vi "getWaveform.vi"(7 "Chn":string, 8 "error in (no error)":errorcluster, 11 "ScopeNi in":refnum<class "ScopeNi.lvclass">) -> (0 "error out":errorcluster, 2 "Waveform Graph":waveform(dbl)(graph), 3 "ScopeNi out":refnum<class "ScopeNi.lvclass">)   [LabVIEW 2023, in "ScopeNi.lvclass"]
doc: "<b>Author:</b> Wolfgang\n<b>Description:</b> Fetches the waveform for the given channel from the scope."
uses:
  ScopeNi.lvclass
  ScopeNi.lvclass/ScopeNi.ctl
  <instrlib>/niScope/Acquire/Fetch/niScope Fetch WDT.vi
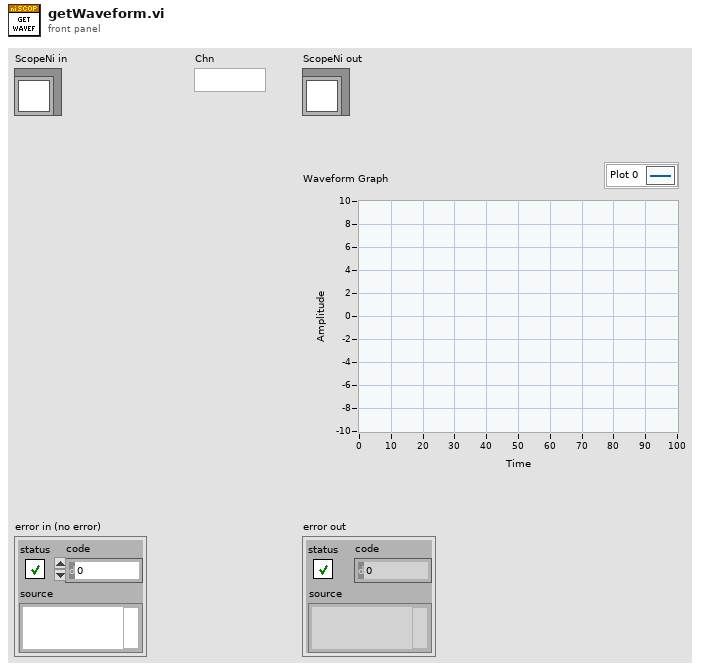
[diagram p1: front panel]
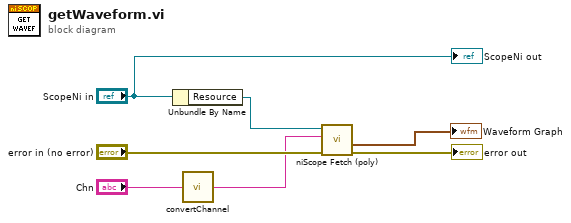
[diagram p0: block diagram]
diagram:
  n1 = Unbundle By Name("ScopeNi in") -> ("Resource"=w5:refnum<k15>)
  n2 = call "convertChannel.vi"("Chn in"="Chn") -> ("Chn out"=w1:string)
  n3 = call-poly <instrlib>:"niScope Fetch (poly).vi"("error in"="error in (no error)", "channels"=w1, "instrument handle"=w5) -> ("error out"=→"error out":errorcluster, "wfm"=→"Waveform Graph":waveform(dbl))  [unwired: 5 in, 2 out]
  "ScopeNi out" <- "ScopeNi in"
